vi "System - Exec Info Host.vi"() -> ()   [LabVIEW 2015, in "ECS-Host.lvlib"]
uses:
  ECS-Host.lvlib
panel:
  out "Storage_Space_Free":u32 caption="[]"
  out "Storage_Space_Used":u32 caption="[]"
  out "Storage_Space":u32 caption="[]"
  out "Largest_Contiguous_Mem":sgl caption="[bytes]"
  out "Memory_Used":sgl caption="[]"
  out "Total_Mem":sgl caption="[]"
  out "CPU_Load_TimeCrit":sgl caption="[]"
  out "CPU_Load":sgl caption="[]"
  out "SCM_Build":string
  out "IP_Address":string
  out "Target_Name":string
  out "SCMInitOK":bool
  out "FPGA_2_Error":bool
  out "FPGA_1_Error":bool
  out "CalFile_Name":string
  in  "SlowSpeedLoopPeriod_Set":u32 caption="[]"
  in  "MainLoopPeriod_Set":u32 caption="[]"
  out "Write_Outputs_Duration":u32 caption="[]"
  out "Control_Duration":u32 caption="[]"
  out "MainLoopPeriod":u32 caption="[]"
  out "Read_Inputs_Duration":u32 caption="[]"
  out "MainLoopDuration":u32 caption="[]"
  # "Note:  Save as default and redeploy\nRT VI to reset main loop period"
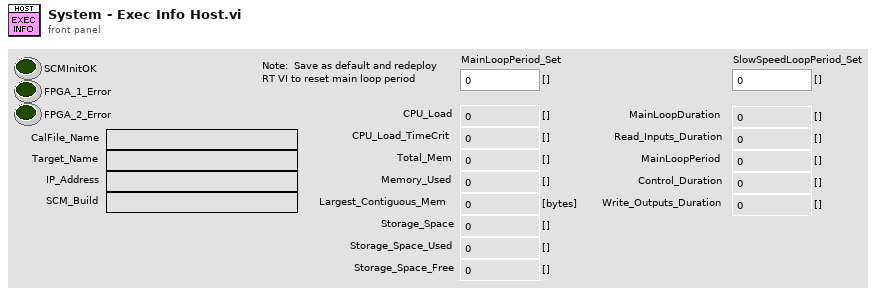
[diagram p1: front panel]
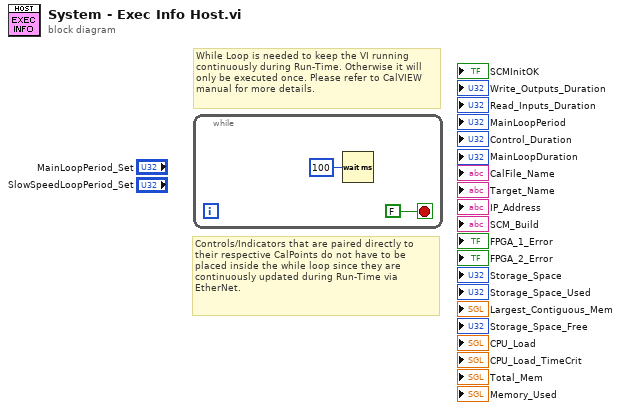
[diagram p0: block diagram]
diagram:
  # "While Loop is needed to keep the VI running\ncontinuously during Run-Time. Otherwise it will only be executed once. Please refer to CalVIEW manual for more details."
  # "Controls/Indicators that are paired directly to their respective CalPoints do not have to be placed inside the while loop since they are continuously updated during Run-Time via EtherNet."
  n1 = while {
    stop <- FALSE stop-if-true
    n2 = Wait (ms)(milliseconds to wait=u32 100) -> ()  [unwired: 1 out]
  }
